vi "Get Software Details (Array).vi"(6 "Trace Component Info (F)":bool, 8 "error in (no error)":errorcluster, 10 "Number of Elements":i32, 11 "Enumerator in":u64) -> (0 "error out":errorcluster, 3 "Software Components":T1[](array[typedef]) {"component type" items=["standard", "hidden", "system", "unknown", "startup", "image", "essential"]})   [LabVIEW 2017, in "nisyscfg.lvlib"]
uses:
  <vilib>/nisyscfg/nisyscfg.lvlib
  <vilib>/nisyscfg/Software 1.2.ctl
  <vilib>/nisyscfg/Component Type.ctl
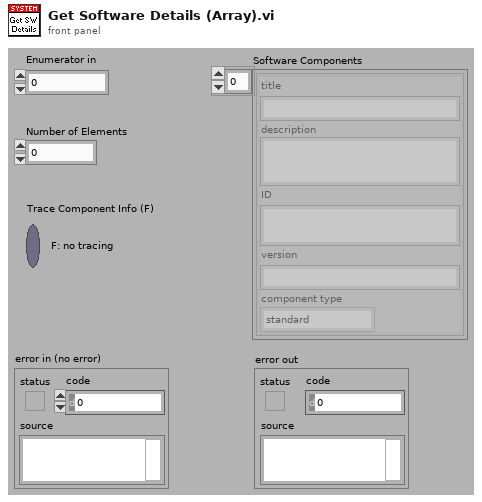
[diagram p1: front panel]
types:
  T1 = typedef "nisyscfg.lvlib/Software 1.2.ctl" = cluster{"title":string, "description":string, "ID":string, "version":string, "component type":T2}
  T2 = typedef "nisyscfg.lvlib/Component Type.ctl" = u32
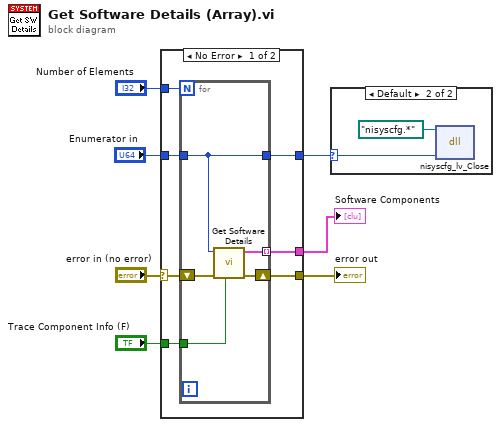
[diagram p0: block diagram]
diagram:
  n1 = case shown="No Error" "error in (no error)" {
    selector: "error in (no error)" -> [w14 w21]
    tunnel: [w13 w21] -> w6
    tunnel: "Enumerator in" -> [w12 w20]
    tunnel: [w11 _] -> w4
    tunnel: "Number of Elements" -> [w10 _]
    tunnel: "Trace Component Info (F)" -> [w9 _]
    tunnel: [w8 w20] -> w1
    frame No Error {
      n2 = for {
        N: w10 -> [_]
        shift-right: [w18] -> w13
        shift-left: w14 -> [w19]
        tunnel: w12 -> [w15]
        tunnel: [w17] -> w11 mode=indexing
        tunnel: w9 -> [w16]
        tunnel: [w15] -> w8
        n3 = call <vilib>:"Get Software Details.vi"("Trace Component Info (F)"=w16, "error in (no error)"=w19, "Enumerator in"=w15) -> ("error out"=w18:errorcluster, "Software Component"=w17:T1)  [unwired: 7 in]
      }
    }
    frame Error {
    }
  }
  "error out" <- w6
  "Software Components" <- w4
  n4 = case shown="Default" w1 {
    selector: w1 -> [_ w22]
    frame 0 {
      # "No need to call Close\non an empty enum."
    }
    frame Default {
      n5 = dll-call lib="nisyscfg.*" fn="nisyscfg_lv_Close" label="Close"(path in=path "nisyscfg.*", "expertsEnum"=w22) -> ()  [unwired: 3 in, 3 out]
    }
  }
